vi "COMn单步调试对话框.vi"() -> ()   [LabVIEW 2016, in "斯坦道CODMn新电路板.lvlib"]
uses:
  <vilib>/Utility/miscctls.llb/LVPointTypeDef.ctl
panel:
  in  "单步调试":T1={"模式选择"=enum."测试模式", "测试模式"={"进样:"=enum."未选择", "偏心轮: "=0, "注射泵:"=enum."未选择", "量: "=5000, "缺液检测"=FALSE, "外设:"={"排液"=FALSE, "搅拌"=FALSE, "风扇"=FALSE, "废液分离"=FALSE}, "加热:"=FALSE, "摄氏度"=0, "阀配置"=0}, "流程模式"={"功能选择"=enum."注入", "阀口选择"=enum."未选择", "外设"={"排液阀"=FALSE, "搅拌"=FALSE, "冷凝风扇"=FALSE, "废液分离阀"=FALSE, "电磁阀1"=FALSE, "电磁阀2"=FALSE, "电磁阀3"=FALSE, "电磁阀4"=FALSE, "电磁阀5"=FALSE, "电磁阀6"=FALSE, "电磁阀7"=FALSE, "顺时针"=FALSE, "逆时针"=FALSE}, "其他"=enum."未选择", "柱塞泵体积μL"=5000, "摄氏度"=0, "加热:"=FALSE}} {"测试模式"."阀配置" items=["三通阀", "排阀"]}
  out "光值8":sgl format="%#.2f"
  out "光值7":sgl format="%#.2f"
  out "光值6":sgl format="%#.2f"
  out "光值5":sgl format="%#.2f"
  out "光值4":sgl format="%#.2f"
  out "光值3":sgl format="%#.2f"
  out "光值2":sgl format="%#.2f"
  out "光值1":sgl format="%#.2f"
  in  "停止":bool
  in  "退出":bool
  in  "启动":bool
  # "CODMn单步调试界面"
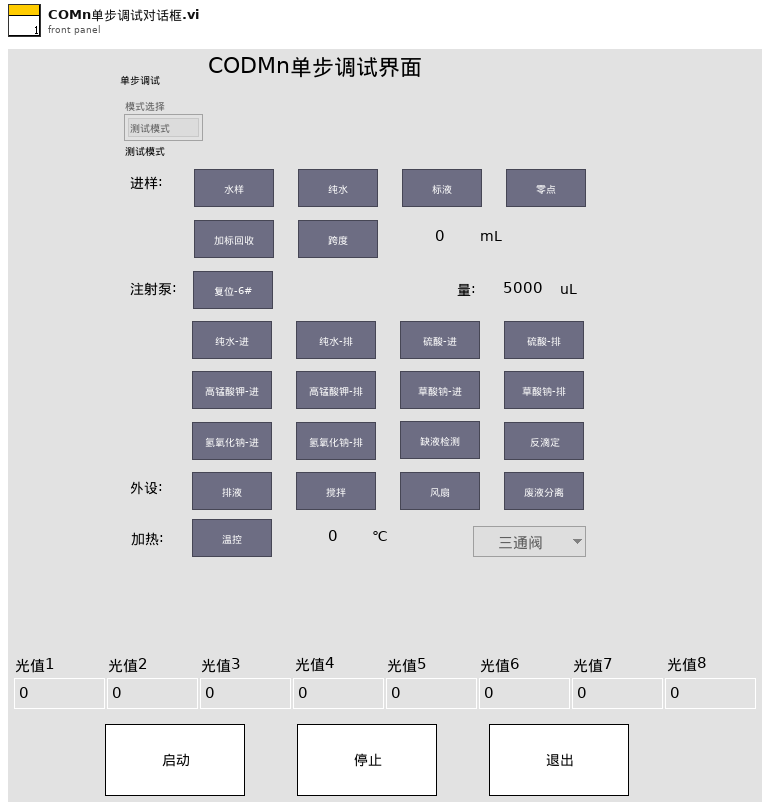
[diagram p1: front panel]
types:
  T1 = cluster{"模式选择":enum16{"测试模式", "流程模式"}, "测试模式":cluster{"进样:":enum32{"未选择", "水样", "纯水", "标液", "零点", "加标回收", "跨度"}, "偏心轮: ":u16, "注射泵:":enum32{"未选择", "纯水-进", "纯水-排", "硫酸-进", "硫酸-排", "复位", "高锰酸钾-进", "高锰酸钾-排", "草酸钠-进", "草酸钠-排", "氢氧化钠-进", "氢氧化钠-排", "反滴定"}, "量: ":u16, "缺液检测":bool, "外设:":cluster{"排液":bool, "搅拌":bool, "风扇":bool, "废液分离":bool}, "加热:":bool, "摄氏度":u16, "阀配置":u8}, "流程模式":cluster{"功能选择":enum32{"等待", "复位", "注入", "注出"}, "阀口选择":enum32{"未选择", "V1", "V2", "V3", "V4", "V5", "V6", "V7", "V8", "V9", "V10", "V11", "V12"}, "外设":cluster{"排液阀":bool, "搅拌":bool, "冷凝风扇":bool, "废液分离阀":bool, "电磁阀1":bool, "电磁阀2":bool, "电磁阀3":bool, "电磁阀4":bool, "电磁阀5":bool, "电磁阀6":bool, "电磁阀7":bool, "顺时针":bool, "逆时针":bool}, "其他":enum32{"未选择", "更新A值", "更新B值", "反滴定"}, "柱塞泵体积μL":u16, "摄氏度":u16, "加热:":bool}}
  T2 = typedef "LVPointTypeDef.ctl" = cluster{"Horizontal":i16, "Vertical":i16}
  T3 = cluster{"泵类型":u8, "阀数量":u8, "纯水通道":u8, "废液通道":u8, "进样速度":u16, "出样速度":u16, "滴定速度":u16, "注射泵保温温度L":u8, "注射泵保温温度H":u8, "注射泵加热超时时间":u16, "是否存在液位检测板":u16, "A值告警下限值":u16, "A值告警上限值":u16, "B值告警下限值":u16, "B值告警上限值":u16, "AB跨度告警值":u16, "阀配置:":u8, "滴定等待时间":u16, "滴定吸光度斜率":dbl, "传感器阈值":u16, "加速模式(速度):":u16}
  T4 = cluster{"阀配置:":u8, "模式选择":enum16{"测试模式", "流程模式"}}
  T5 = cluster{"数组":u16[], "模式选择":enum16{"测试模式", "流程模式"}}
  T6 = cluster{"系统时间":timestamp, "工作状态":u16, "测量模式":enum16{"待机", "连续模式", "周期模式", "定点模式", "受控模式", "手动模式"}, "告警代码":u16, "故障代码":u16, "日志代码":u16, "软件版本":u16, "A":sgl, "B":sgl, "K":sgl, "当前滴定数":sgl, "T":sgl, "H":sgl, "id":u16, "flowid":u16, "量程":u16, "加热实时温度":sgl, "当前ORP值":sgl, "运行时间":sgl, "当前步骤剩余时间":sgl, "结束滴定数":sgl, "注射泵保温温度":sgl, "匹配滴定数X0":u16, "X^2":sgl, "X":sgl, "B 2":sgl, "光值1":sgl, "光值2":sgl, "光值3":sgl, "光值4":sgl, "光值5":sgl, "光值6":sgl, "光值7":sgl, "光值8":sgl}
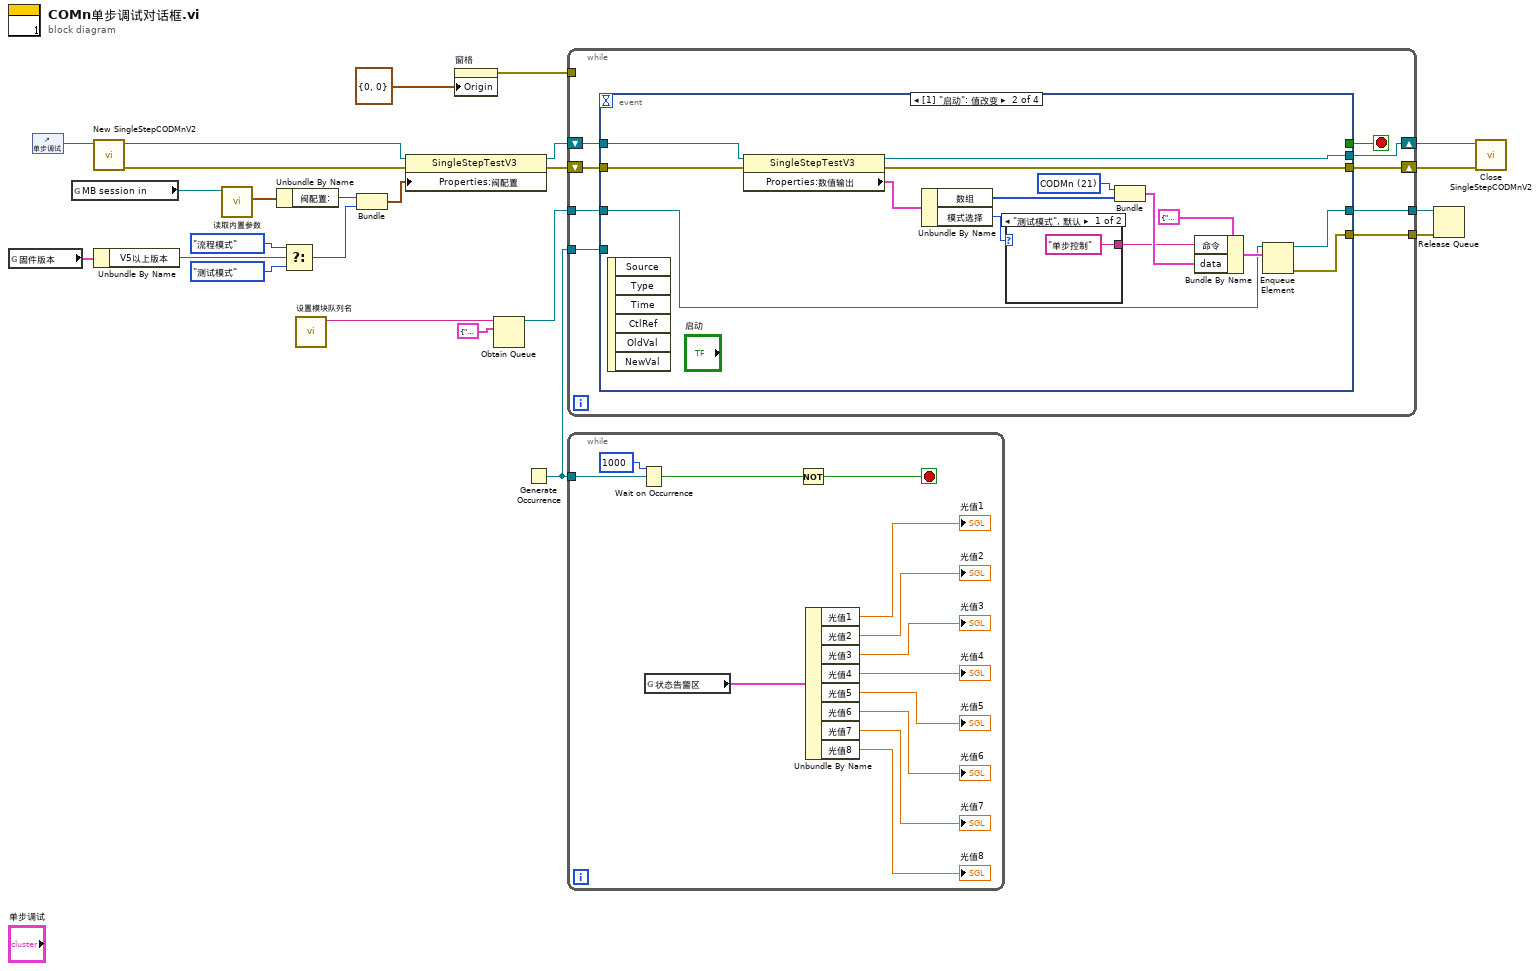
[diagram p0: block diagram]
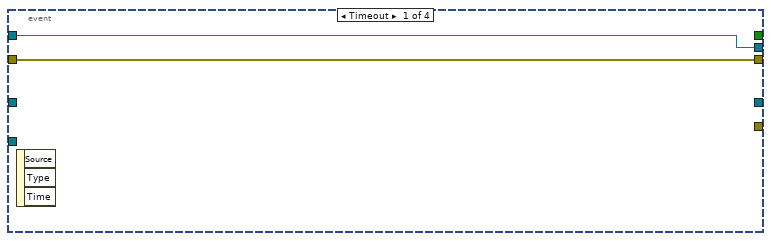
[diagram p2: hidden frame]
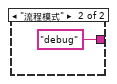
[diagram p3: hidden frame]
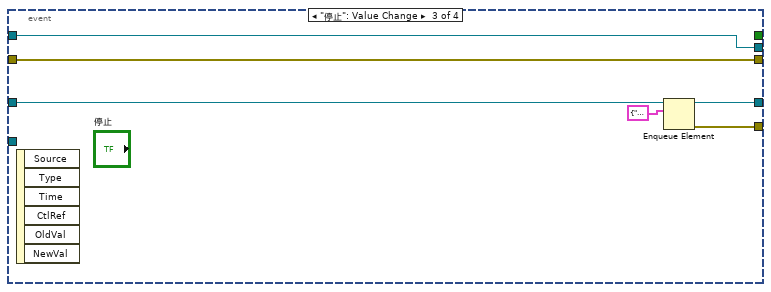
[diagram p4: hidden frame]
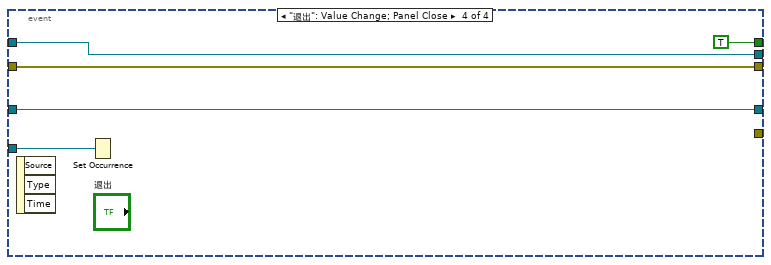
[diagram p5: hidden frame]
diagram:
  n1 = global read "VARCODMn全局变量.vi" "固件版本"() -> (w2:cluster{"V5以上版本":bool, "版本号":dbl})
  n2 = control-ref of="单步调试"() -> (w3:refnum<vi>)
  n3 = global read "VARCODMn全局变量.vi" "MB session in"() -> (w18:refnum<class "MB_Master.lvclass">)
  n4 = call "New SingleStepCODMnV2.vi"("Reference"=w3) -> ("error out"=w9:errorcluster, "SingleStepTestV3 out"=w14:refnum<class "SingleStepCODMnV2.lvclass">)  [unwired: 9 in]
  n5 = Unbundle By Name(w2) -> ("V5以上版本"=w1:bool)
  n6 = call "读取内置参数.vi"("MB session in"=w18) -> ("外设配置"=w17:T3)  [unwired: 6 in, 4 out]
  n7 = Unbundle By Name(w17) -> ("阀配置:"=w13:u8)
  n8 = Select(t=enum16{"测试模式", "流程模式"}."流程模式" ("模式选择"), s=w1, f=enum16{"测试模式", "流程模式"}."测试模式" ("模式选择")) -> (s? t:f=w4:enum16{"测试模式", "流程模式"})
  n9 = call "设置模块队列名.vi"() -> ("Msg"=w15:string)  [unwired: 11 in]
  n10 = Bundle("阀配置:"=w13, "模式选择"=w4) -> (w12:T4)  [unwired: 1 in]
  n11 = property class="SingleStepTestV3"(reference=w14, error in=w9, "Properties:阀配置"=w12) -> (reference out=w11:refnum<class "SingleStepCODMnV2.lvclass">, error out=w10:errorcluster)
  n12 = property on="窗格" class="Pane"("Origin"=T2 {"Horizontal"=0, "Vertical"=0} ("原点")) -> (error out=w20:errorcluster)  [unwired: 2 in, 1 out]
  n13 = Obtain Queue(name (unnamed)=w15, element data type=cluster{"命令":string, "data":variant} {"命令"="", "data"=variant}) -> (queue out=w23:refnum<queue>)  [unwired: 3 in, 2 out]
  n14 = Generate Occurrence() -> (w16:refnum<k4>)
  n15 = while {
    tunnel: w23 -> [w32]
    tunnel: [w31] -> w22
    tunnel: [w30] -> w21
    tunnel: w20 -> [_]
    tunnel: w16 -> [w29]
    shift-right: [w27] -> w8
    shift-left: w11 -> [w28]
    shift-right: [w26] -> w7
    shift-left: w10 -> [w25]
    stop <- w33 stop-if-true
    n16 = event shown="[1] \"启动\": 值改变" {
      selector: _ -> [_ _ _ _]
      dyn-events: _ -> [_ _ _ _]
      timeout: _ -> [_ _ _ _]
      tunnel: [_ _ _ TRUE] -> w33
      tunnel: w32 -> [_ w46 w57 w62]
      tunnel: [_ w45 w56 w62] -> w31
      tunnel: [_ w44 w55 _] -> w30
      tunnel: w29 -> [_ _ _ w61]
      tunnel: w28 -> [w35 w40 w54 w60]
      tunnel: [w35 w38 w54 w60] -> w27
      tunnel: [w34 w37 w53 w59] -> w26
      tunnel: w25 -> [w34 w36 w53 w59]
      event Timeout {
        n17 = event-data() -> ()  [unwired: 1 in, 3 out]
      }
      event "启动": Value Change {
        w48 = u16 21 items=["CODMn"=21, "总磷"=1, "氨氮"=3] ("站号")
        n18 = event-data() -> ()  [unwired: 1 in, 6 out]
        n19 = property class="SingleStepTestV3"(reference=w40, error in=w36) -> (reference out=w38:refnum<class "SingleStepCODMnV2.lvclass">, error out=w37:errorcluster, "Properties:数值输出"=w39:T5)
        n20 = Unbundle By Name(w39) -> ("数组"=w43:u16[], "模式选择"=w42:enum16{"测试模式", "流程模式"})
        n21 = case shown="\"测试模式\", 默认" w42 {
          tunnel: ["单步控制" ("命令") "debug" ("命令")] -> w41
          frame "测试模式", Default {
          }
          frame "流程模式" {
          }
        }
        n22 = Bundle("站号"=w48, "数组"=w43) -> (w47:cluster{"站号":u16, "数组":u16[]})  [unwired: 1 in]
        n23 = Bundle By Name(cluster=cluster{"命令":string, "data":variant} {"命令"="", "data"=variant} ("元素"), "命令"=w41, "data"=w47) -> (w49:cluster{"命令":string, "data":variant})
        n24 = Enqueue Element(queue=w46, element=w49) -> (queue out=w45:refnum<queue>, error out=w44:errorcluster)  [unwired: 2 in, 1 out]
      }
      event "停止": Value Change {
        n25 = event-data() -> ()  [unwired: 1 in, 6 out]
        n26 = Enqueue Element(queue=w57, element=cluster{"命令":string, "data":variant} {"命令"="启动", "data"=variant(cluster{"站号":u16, "控制命令":u16[]} {"站号"=21, "控制命令"=[2816]})} ("启动命令")) -> (queue out=w56:refnum<queue>, error out=w55:errorcluster)  [unwired: 2 in, 1 out]
      }
      event "退出": Value Change; Panel Close {
        n27 = event-data() -> ()  [unwired: 1 in, 3 out]
        n28 = Set Occurrence(w61) -> ()
      }
    }
  }
  n29 = while {
    tunnel: w16 -> [w64]
    stop <- w66 stop-if-true
    n30 = Wait on Occurrence(2:w64, 3:1000 ("毫秒超时(-1)")) -> (0:w67:bool)  [unwired: 1 in]
    n31 = global read "VARCODMn全局变量.vi" "状态告警区"() -> (w76:T6)
    n32 = Not(x=w67) -> (.not. x?=w66:bool)
    n33 = Unbundle By Name(w76) -> ("光值1"=→"光值1":sgl, "光值2"=→"光值2":sgl, "光值3"=→"光值3":sgl, "光值4"=→"光值4":sgl, "光值5"=→"光值5":sgl, "光值6"=→"光值6":sgl, "光值7"=→"光值7":sgl, "光值8"=→"光值8":sgl)
  }
  n34 = Release Queue(queue=w22, error in (no error)=w21) -> ()  [unwired: 1 in, 3 out]
  n35 = call "Close SingleStepCODMnV2.vi"("error in (no error)"=w7, "SingleStepTestV3 in"=w8) -> ()  [unwired: 9 in, 1 out]
